vi "Configuration File.vi"(8 "error in (no error)":errorcluster, 11 "Node Ptr":T3 format="%.0x") -> (0 "error out":errorcluster)   [LabVIEW 2020, in "AIM ARINC 664 System Explorer.lvlib" / "Implementation.lvlib"]
uses:
  Implementation.lvlib
  <vilib>/NI VeriStand/Custom Device API/Custom Device Item Ref.ctl
  Types/Path Control.ctl
  Types/Browse Button.ctl
  Types/Configuration File Page Data.ctl
  <vilib>/NI VeriStand/Custom Device API/Custom Device API.lvlib
  Scripting/AIM ARINC 664 Scripting.lvlib
  <vilib>/NI VeriStand/Custom Device Tools/Custom Device Utility Library/Custom Device Utility Library.lvlib
panel:
  in  "Payload":T1
  in  "Parameters":T1
  in  "Refresh":bool
  in  "SHDocVw.IWebBrowser":refnum<k7>(container)
  in  "General Header":cluster{"Section Name":string}={"Section Name"="General Custom Device Settings"}
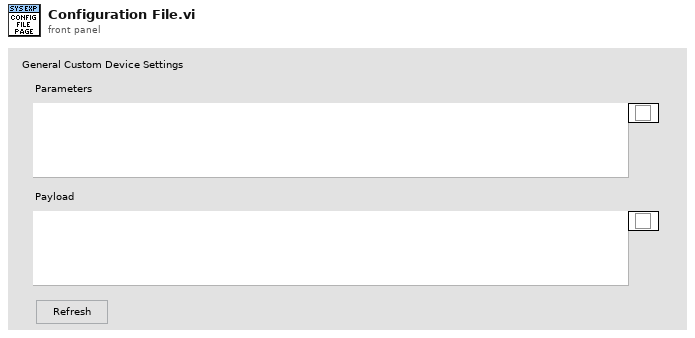
[diagram p1: front panel]
types:
  T1 = typedef "AIM ARINC 664 System Explorer.lvlib/Implementation.lvlib/Path Control.ctl" = cluster{"file path":path, "Browse":T2}
  T2 = typedef "AIM ARINC 664 System Explorer.lvlib/Implementation.lvlib/Browse Button.ctl" = bool
  T3 = typedef "Custom Device API.lvlib/Custom Device Item Ref.ctl" = u64
  T4 = typedef "AIM ARINC 664 System Explorer.lvlib/Implementation.lvlib/Configuration File Page Data.ctl" = cluster{"Parameters":T1, "most recent configuration path":path, "custom device ref":T3, "MD5":string, "configuration path ctl ref":refnum<vi>, "CD scripted?":bool}
  T5 = typedef "Custom Device API.lvlib/Custom Device Commands.ctl" = enum16{"Default", "Item renamed", "Shutdown", "Dynamic button pressed"}
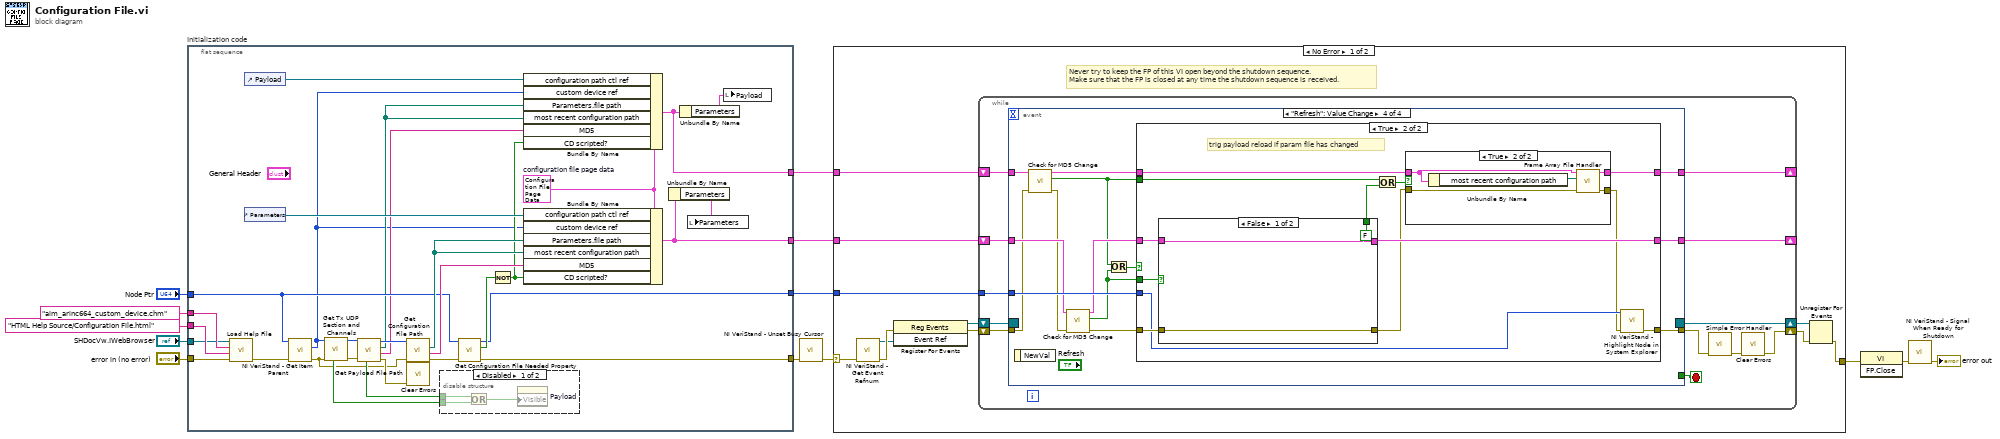
[diagram p0: block diagram]
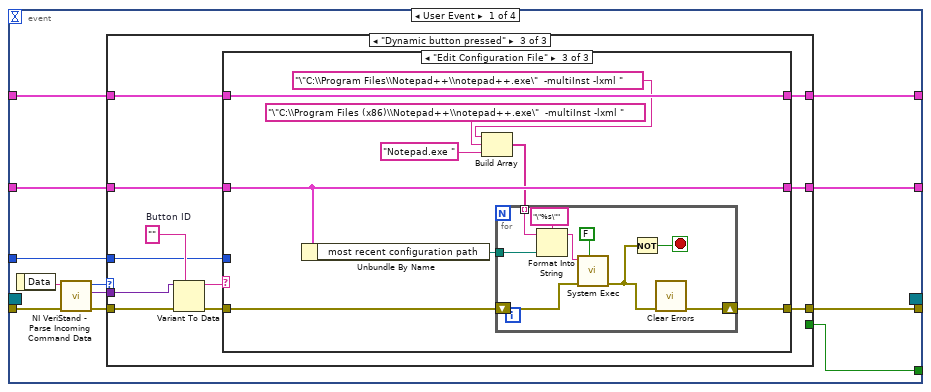
[diagram p3: hidden frame]
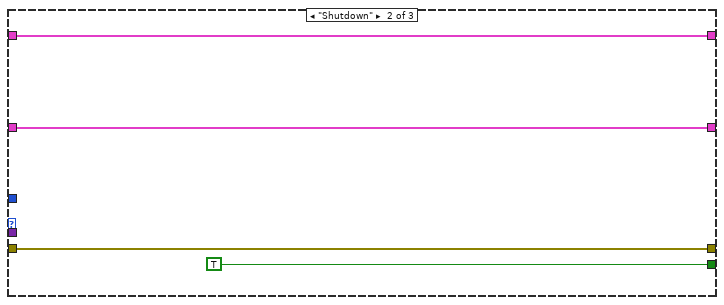
[diagram p5: hidden frame]
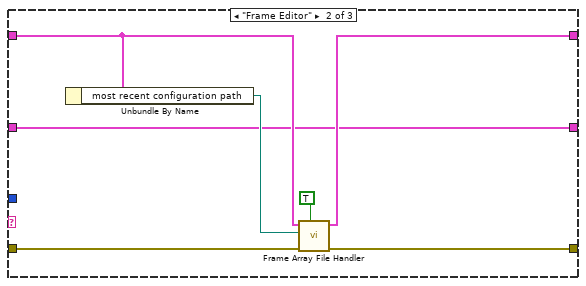
[diagram p7: hidden frame]
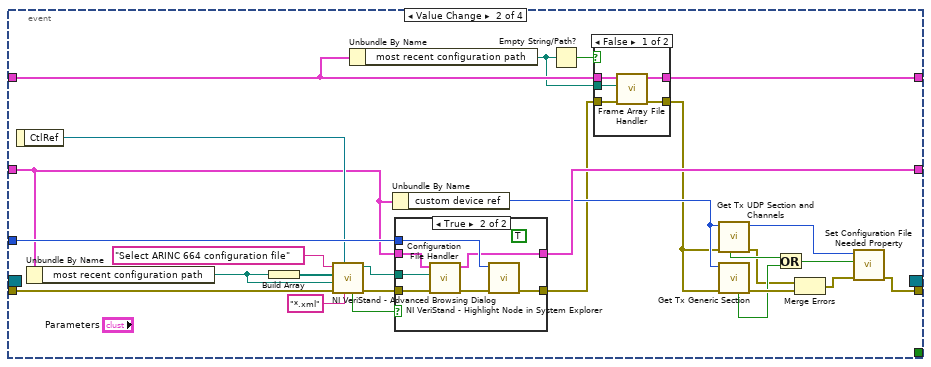
[diagram p8: hidden frame]
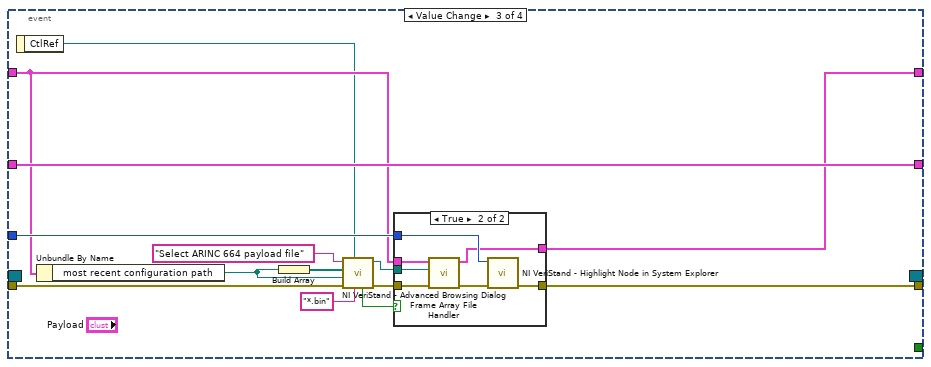
[diagram p11: hidden frame]
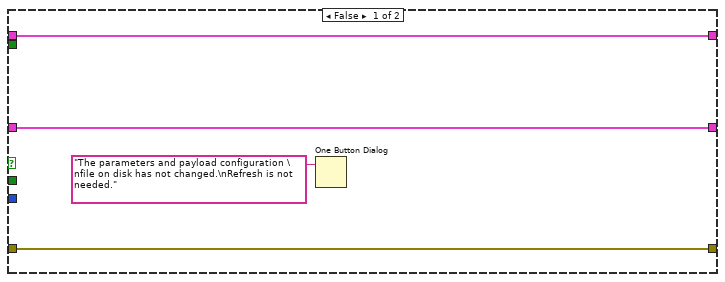
[diagram p13: hidden frame]
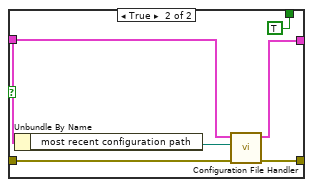
[diagram p15: hidden frame]
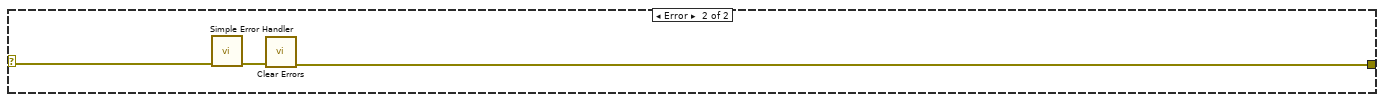
[diagram p16: hidden frame]
diagram:
  n1 = flat-sequence "Initialization code" {
    tunnel: "error in (no error)" -> [w43]
    tunnel: "Node Ptr" -> [w30]
    tunnel: [w32] -> w9
    tunnel: "SHDocVw.IWebBrowser" -> [w39]
    tunnel: "HTML Help Source/Configuration File.html" ("HTML File") -> [w40]
    tunnel: "aim_arinc664_custom_device.chm" ("CD_CHM_FileName") -> [w41]
    tunnel: [w36] -> w3
    tunnel: [w29] -> w2
    tunnel: [w21] -> w1
    frame #0 {
      w27 = T4 {"Parameters"={"file path"=path "", "Browse"=FALSE}, "most recent configuration path"=path "", "custom device ref"=0, "MD5"="", "configuration path ctl ref"=refnum, "CD scripted?"=FALSE}  # configuration file page data
      n2 = call "Load Help File.vi"("error in (no error)"=w43, "HTML File to Load"=w40, "Main CHM File"=w41, "Browser"=w39) -> ("error out"=w42:errorcluster)  [unwired: 6 in, 1 out]
      n3 = control-ref of="Payload"() -> (w23:refnum<vi>)
      n4 = control-ref of="Parameters"() -> (w33:refnum<vi>)
      n5 = call <vilib>:"NI VeriStand - Get Item Parent.vi"("error in (no error)"=w42, "Item Ref in"=w30) -> ("error out"=w14:errorcluster, "Parent Ref"=w18:T3)  [unwired: 6 in, 2 out]
      n6 = call "Get Tx UDP Section and Channels.vi"("error in"=w14, "custom device ref in"=w18) -> ("error out"=w16:errorcluster, "custom device ref out"=w19:T3, "session found?"=w17:bool)  [unwired: 4 in, 3 out]
      n7 = call "Get Payload File Path.vi"("error in"=w16, "custom device ref in"=w19) -> ("error out"=w15:errorcluster, "MD5 checksum"=w25:string, "frame array file path"=w26:path, "custom device ref out"=w28:T3, "found Tx Gen?"=w20:bool)  [unwired: 4 in, 1 out]
      n8 = call "Get Configuration File Path.vi"("error in"=w14, "custom device ref in"=w28) -> ("error out"=w38:errorcluster, "MD5 checksum"=w37:string, "configuration file path"=w35:path)  [unwired: 5 in, 2 out]
      n9 = call <vilib>:"Clear Errors.vi"("error in (no error)"=w15) -> ()  [unwired: 5 in, 2 out]
      n10 = disable-structure shown="Disabled" {
        disable-tunnel: w20 -> [w46 _]
        disable-tunnel: w17 -> [w44 _]
        frame Disabled {
          n11 = Or(x=w46, y=w44) -> (x .or. y?=w45:bool)
          n12 = property on="Payload" class="Clust (strict)"("Visible"=w45) -> ()  [unwired: 2 in, 2 out]
        }
        frame Enabled {
        }
      }
      n13 = call "Get Configuration File Needed Property.vi"("error in"=w38, "configuration file section ref in"=w30) -> ("error out"=w32:errorcluster, "needed?"=w31:bool, "configuration file section ref out"=w29:T3)  [unwired: 7 in]
      n14 = Not(x=w31) -> (.not. x?=w24:bool)
      n15 = Bundle By Name(cluster=w27, "configuration path ctl ref"=w23, "custom device ref"=w18, "Parameters.file path"=w26, "most recent configuration path"=w26, "MD5"=w25, "CD scripted?"=w24) -> (w21:T4)
      n16 = Bundle By Name(cluster=w27, "configuration path ctl ref"=w33, "custom device ref"=w18, "Parameters.file path"=w35, "most recent configuration path"=w35, "MD5"=w37, "CD scripted?"=w24) -> (w36:T4)
      n17 = Unbundle By Name(w36) -> ("Parameters"=w34:T1)
      n18 = Unbundle By Name(w21) -> ("Parameters"=w22:T1)
      n19 = local write "Parameters"(w34) -> ()
      n20 = local write "Payload"(w22) -> ()
    }
  }
  n21 = call <vilib>:"NI VeriStand - Unset Busy Cursor.vi"("error in (no error)"=w9) -> ("error out"=w8:errorcluster)  [unwired: 10 out]
  n22 = case shown="No Error" w8 {
    selector: w8 -> [w49 w243]
    tunnel: [w54 w241] -> w13
    tunnel: w2 -> [w50 _]
    tunnel: w3 -> [w48 _]
    tunnel: w1 -> [w47 _]
    frame No Error {
      # "Never try to keep the FP of this VI open beyond the shutdown sequence.\nMake sure that the FP is closed at any time the shutdown sequence is received."
      n23 = call <vilib>:"NI VeriStand - Get Event Refnum.vi"("error in (no error)"=w49) -> ("error out"=w57:errorcluster, "Event Ref"=w53:refnum<user-event>)  [unwired: 9 out]
      n24 = register-events(error in=w57, w53) -> (reference out=w51:refnum<event-registration>, error out=w52:errorcluster)  [unwired: 1 in]
      n25 = while {
        tunnel: w50 -> [w65]
        shift-right: [w62] -> w55
        shift-left: w52 -> [w68]
        shift-right: [w69] -> w56
        shift-left: w51 -> [w67]
        shift-right: [w60] -> _
        shift-left: w48 -> [w61]
        shift-right: [w58] -> _
        shift-left: w47 -> [w59]
        stop <- w66 stop-if-true
        n26 = event shown="[3] \"Refresh\": Value Change" {
          selector: w67 -> [_ _ _ _]
          dyn-events: [_ _ _ _] -> w69
          timeout: _ -> [_ _ _ _]
          tunnel: w68 -> [w81 w154 w179 w201]
          tunnel: [w77 _ _ _] -> w66
          tunnel: [w76 w129 w176 w206] -> w64
          tunnel: w65 -> [w75 w146 w175 w205]
          tunnel: w61 -> [w71 w143 w184 w203]
          tunnel: [w70 w145 w184 w207] -> w60
          tunnel: w59 -> [w73 w139 w173 w199]
          tunnel: [w72 w137 w172 w197] -> w58
          event User Event {
            n27 = event-data() -> ("Data"=w80:string)  [unwired: 1 out]
            n28 = call <vilib>:"NI VeriStand - Parse Incoming Command Data.vi"("error in (no error)"=w81, "Incoming data"=w80) -> ("error out"=w79:errorcluster, "Outgoing data"=w74:variant, "Action"=w78:T5)  [unwired: 7 out]
            n29 = case shown="\"Dynamic button pressed\"" w78 {
              tunnel: w79 -> [w84 w87 w99]
              tunnel: [_ TRUE _] -> w77
              tunnel: [w84 w87 w94] -> w76
              tunnel: w75 -> [_ _ w92]
              tunnel: w74 -> [_ _ w98]
              tunnel: w73 -> [w83 w86 w93]
              tunnel: [w83 w86 w91] -> w72
              tunnel: w71 -> [w82 w85 w90]
              tunnel: [w82 w85 w89] -> w70
              frame "Default", Default {
              }
              frame "Shutdown" {
              }
              frame "Dynamic button pressed" {
                w97 = ""  # Button ID
                n30 = Variant To Data(error in=w99, type=w97, Variant=w98) -> (data=w96:string, error out=w95:errorcluster)
                n31 = case shown="\"Edit Configuration File\"" w96 {
                  tunnel: w95 -> [w102 w109 w116]
                  tunnel: [w102 w107 w115] -> w94
                  tunnel: w93 -> [w101 w106 w118]
                  tunnel: w92 -> [_ _ _]
                  tunnel: [w101 w108 w118] -> w91
                  tunnel: w90 -> [w100 w104 w117]
                  tunnel: [w100 w104 w117] -> w89
                  frame Default {
                  }
                  frame "Frame Editor" {
                    n32 = Unbundle By Name(w106) -> ("most recent configuration path"=w105:path)
                    n33 = call "Frame Array File Handler.vi"("launch utility?"=TRUE, "error in"=w109, "selected frame array file"=w105, "configuration file page data"=w106) -> ("error out"=w107:errorcluster, "configuration file page data out"=w108:T4)  [unwired: 6 in]
                  }
                  frame "Edit Configuration File" {
                    n34 = Unbundle By Name(w117) -> ("most recent configuration path"=w114:path)
                    n35 = Build Array("\"C:\\Program Files\\Notepad++\\notepad++.exe\"  -multiInst -lxml " ("format string"), "\"C:\\Program Files (x86)\\Notepad++\\notepad++.exe\"  -multiInst -lxml " ("format string"), "Notepad.exe " ("format string")) -> (w112:string[])
                    n36 = for {
                      tunnel: w114 -> [w126]
                      tunnel: w112 -> [w121] mode=indexing
                      shift-right: [w124] -> w115
                      shift-left: w116 -> [w127]
                      stop <- w123 stop-if-true
                      n37 = Format Into String(format string="\"%s\"", initial string=w121, w126) -> (resulting string=w125:string)  [unwired: 1 in, 1 out]
                      n38 = call <vilib>:"System Exec.vi"("wait until completion? (T)"=FALSE, "error in (no error)"=w127, "command line"=w125) -> ("error out"=w122:errorcluster)  [unwired: 5 in, 3 out]
                      n39 = Not(x=w122) -> (.not. x?=w123:bool)
                      n40 = call <vilib>:"Clear Errors.vi"("error in (no error)"=w122) -> ("error out"=w124:errorcluster)  [unwired: 5 in, 1 out]
                    }
                  }
                }
              }
            }
          }
          event Value Change {
            n41 = event-data() -> ("CtlRef"=w144:refnum<vi>)  [unwired: 1 out]
            n42 = Unbundle By Name(w143) -> ("most recent configuration path"=w151:path)
            n43 = Build Array(w151) -> (w152:path[])
            n44 = call <vilib>:"NI VeriStand - Advanced Browsing Dialog.vi"("File Pattern"="*.xml", "CtlRef"=w144, "error in (no error)"=w154, "Most recent path"=w151, "Paths"=w152, "Dialog Title"="Select ARINC 664 configuration file") -> ("error out"=w148:errorcluster, "Selected file"=w147:path, "Valid?"=w149:bool)  [unwired: 2 in, 1 out]
            n45 = Unbundle By Name(w139) -> ("most recent configuration path"=w138:path)
            n46 = Unbundle By Name(w143) -> ("custom device ref"=w141:T3)
            n47 = case shown="True" w149 {
              tunnel: w148 -> [w162 w170]
              tunnel: w147 -> [_ w169]
              tunnel: w143 -> [w163 w168]
              tunnel: [w162 w166] -> w136
              tunnel: w146 -> [_ w165]
              tunnel: [w163 w164] -> w145
              frame False {
              }
              frame True {
                (unwired) TRUE
                n48 = call "Configuration File Handler.vi"("error in"=w170, "selected configuration file"=w169, "configuration file page data"=w168) -> ("error out"=w167:errorcluster, "configuration file page data out"=w164:T4)  [unwired: 7 in]
                n49 = call <vilib>:"NI VeriStand - Highlight Node in System Explorer.vi"("error in (no error)"=w167, "Item Ref in"=w165) -> ("error out"=w166:errorcluster)  [unwired: 8 in, 1 out]
              }
            }
            n50 = Empty String/Path?(string/path=w138) -> (empty?=w140:bool)
            n51 = case shown="False" w140 {
              tunnel: w139 -> [w159 w161]
              tunnel: w138 -> [w158 _]
              tunnel: [w157 w161] -> w137
              tunnel: w136 -> [w156 w160]
              tunnel: [w155 w160] -> w135
              frame False {
                n52 = call "Frame Array File Handler.vi"("error in"=w156, "selected frame array file"=w158, "configuration file page data"=w159) -> ("error out"=w155:errorcluster, "configuration file page data out"=w157:T4)  [unwired: 7 in]
              }
              frame True {
              }
            }
            n53 = call "Get Tx UDP Section and Channels.vi"("error in"=w135, "custom device ref in"=w141) -> ("error out"=w128:errorcluster, "custom device ref out"=w131:T3, "session found?"=w132:bool)  [unwired: 4 in, 3 out]
            n54 = call "Get Tx Generic Section.vi"("error in"=w135, "Parent section Ref in"=w141) -> ("error out"=w142:errorcluster, "found?"=w134:bool)  [unwired: 6 in, 2 out]
            n55 = Or(x=w132, y=w134) -> (x .or. y?=w133:bool)
            n56 = Merge Errors(w128, w142) -> (w130:errorcluster)
            n57 = call "Set Configuration File Needed Property.vi"("error in"=w130, "needed?"=w133, "custom device ref in"=w131) -> ("error out"=w129:errorcluster)  [unwired: 7 in, 1 out]
          }
          event Value Change {
            n58 = event-data() -> ("CtlRef"=w171:refnum<vi>)  [unwired: 1 out]
            n59 = Unbundle By Name(w173) -> ("most recent configuration path"=w181:path)
            n60 = Build Array(w181) -> (w182:path[])
            n61 = call <vilib>:"NI VeriStand - Advanced Browsing Dialog.vi"("File Pattern"="*.bin", "CtlRef"=w171, "error in (no error)"=w179, "Most recent path"=w181, "Paths"=w182, "Dialog Title"="Select ARINC 664 payload file") -> ("error out"=w177:errorcluster, "Selected file"=w174:path, "Valid?"=w178:bool)  [unwired: 2 in, 1 out]
            n62 = case shown="True" w178 {
              tunnel: w177 -> [w185 w193]
              tunnel: w174 -> [_ w192]
              tunnel: w173 -> [w186 w191]
              tunnel: [w185 w189] -> w176
              tunnel: w175 -> [_ w188]
              tunnel: [w186 w187] -> w172
              frame False {
              }
              frame True {
                n63 = call "Frame Array File Handler.vi"("error in"=w193, "selected frame array file"=w192, "configuration file page data"=w191) -> ("error out"=w190:errorcluster, "configuration file page data out"=w187:T4)  [unwired: 7 in]
                n64 = call <vilib>:"NI VeriStand - Highlight Node in System Explorer.vi"("error in (no error)"=w190, "Item Ref in"=w188) -> ("error out"=w189:errorcluster)  [unwired: 8 in, 1 out]
              }
            }
          }
          event "Refresh": Value Change {
            n65 = event-data() -> ()  [unwired: 2 out]
            n66 = call "Check for MD5 Change.vi"("error in"=w201, "configuration file page data"=w199) -> ("error out"=w196:errorcluster, "MD5 change?"=w195:bool, "configuration file page data out"=w198:T4)  [unwired: 7 in]
            n67 = call "Check for MD5 Change.vi"("error in"=w196, "configuration file page data"=w203) -> ("error out"=w204:errorcluster, "MD5 change?"=w194:bool, "configuration file page data out"=w202:T4)  [unwired: 7 in]
            n68 = Or(x=w195, y=w194) -> (x .or. y?=w200:bool)
            n69 = case shown="True" w200 {
              tunnel: w202 -> [w211 w223]
              tunnel: [w211 w224] -> w207
              tunnel: w204 -> [w209 w222]
              tunnel: [w209 w216] -> w206
              tunnel: w205 -> [_ w221]
              tunnel: w198 -> [w208 w219]
              tunnel: [w208 w220] -> w197
              tunnel: w195 -> [_ w214]
              tunnel: w194 -> [_ w215]
              frame False {
                n70 = One Button Dialog(message="The parameters and payload configuration \nfile on disk has not changed.\nRefresh is not needed.") -> ()  [unwired: 1 in, 1 out]
              }
              frame True {
                # "trig payload reload if param file has changed"
                n71 = case shown="False" w215 {
                  tunnel: [w233 w240] -> w224
                  tunnel: w223 -> [w233 w238]
                  tunnel: w222 -> [w234 w237]
                  tunnel: [w234 w236] -> w218
                  tunnel: [FALSE TRUE] -> w212
                  frame False {
                  }
                  frame True {
                    n72 = Unbundle By Name(w238) -> ("most recent configuration path"=w239:path)
                    n73 = call "Configuration File Handler.vi"("error in"=w237, "selected configuration file"=w239, "configuration file page data"=w238) -> ("error out"=w236:errorcluster, "configuration file page data out"=w240:T4)  [unwired: 7 in]
                  }
                }
                n74 = Or(x=w214, y=w212) -> (x .or. y?=w213:bool)
                n75 = case shown="True" w213 {
                  tunnel: [w226 w230] -> w220
                  tunnel: w219 -> [w226 w229]
                  tunnel: w218 -> [w225 w228]
                  tunnel: [w225 w227] -> w217
                  frame False {
                  }
                  frame True {
                    n76 = Unbundle By Name(w229) -> ("most recent configuration path"=w231:path)
                    n77 = call "Frame Array File Handler.vi"("error in"=w228, "selected frame array file"=w231, "configuration file page data"=w229) -> ("error out"=w227:errorcluster, "configuration file page data out"=w230:T4)  [unwired: 7 in]
                  }
                }
                n78 = call <vilib>:"NI VeriStand - Highlight Node in System Explorer.vi"("error in (no error)"=w217, "Item Ref in"=w221) -> ("error out"=w216:errorcluster)  [unwired: 8 in, 1 out]
              }
            }
          }
        }
        n79 = call <vilib>:"Simple Error Handler.vi"("error in (no error)"=w64) -> ("error out"=w63:errorcluster)  [unwired: 1 in, 7 out]
        n80 = call <vilib>:"Clear Errors.vi"("error in (no error)"=w63) -> ("error out"=w62:errorcluster)  [unwired: 1 in, 5 out]
      }
      n81 = Unregister For Events(event registration refnum=w56, error in=w55) -> (error out=w54:errorcluster)
    }
    frame Error {
      n82 = call <vilib>:"Simple Error Handler.vi"("error in (no error)"=w243) -> ("error out"=w242:errorcluster)  [unwired: 1 in, 7 out]
      n83 = call <vilib>:"Clear Errors.vi"("error in (no error)"=w242) -> ("error out"=w241:errorcluster)  [unwired: 1 in, 5 out]
    }
  }
  n84 = invoke class="VI" method="FP.Close"(error in=w13) -> (error out=w12:errorcluster)  [unwired: 2 in, 2 out]
  n85 = call <vilib>:"NI VeriStand - Signal When Ready for Shutdown.vi"("error in (no error)"=w12) -> ("error out"=→"error out":errorcluster)  [unwired: 10 out]
